vi "Configure Limit.vi"(4 "Lower Limit":dbl, 5 "Upper Limit":dbl, 6 "Enable Lower Limit (T: On)":bool=TRUE, 7 "Enable Upper Limit (T: On)":bool=TRUE, 8 "error in (no error)":errorcluster, 11 "VISA resource name":refnum<visa-resource-name>) -> (0 "error out":errorcluster, 3 "VISA resource name out":refnum<visa-resource-name>)   [LabVIEW 2019, in "Pendulum CNT90.lvlib"]
doc: "Turns On/Off the limit-monitoring calculations and the chacking against the lower or upper limit. And configures lower and upper limit."
uses:
  Pendulum CNT90.lvlib
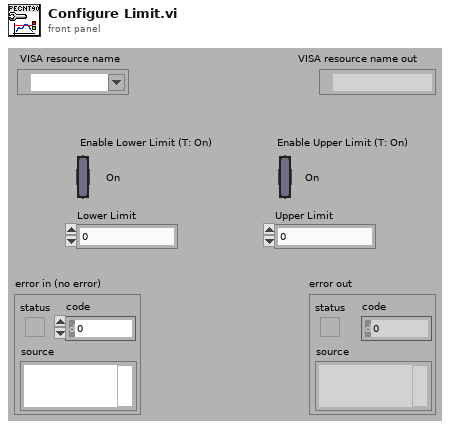
[diagram p1: front panel]
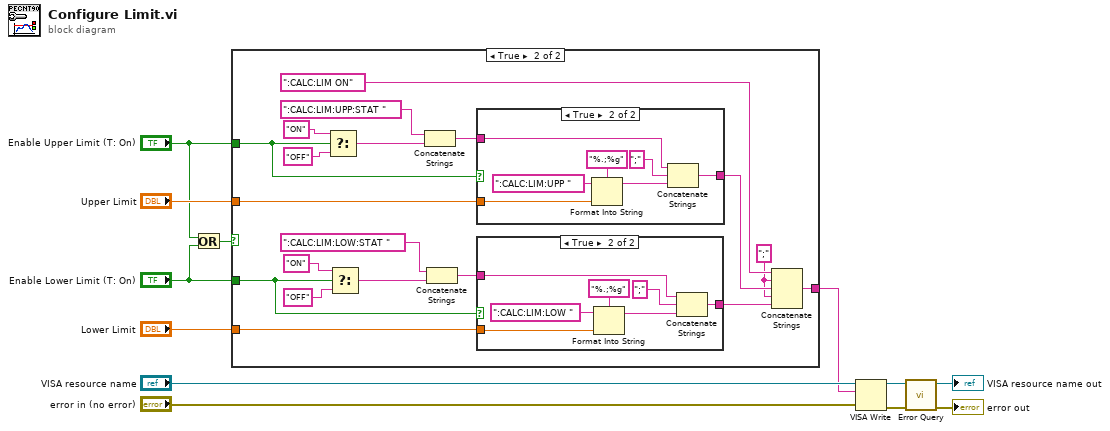
[diagram p0: block diagram]
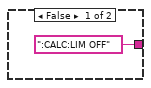
[diagram p2: hidden frame]
diagram:
  n1 = Or(x="Enable Upper Limit (T: On)", y="Enable Lower Limit (T: On)") -> (x .or. y?=w3:bool)
  n2 = case shown="True" w3 {
    tunnel: "Upper Limit" -> [_ w32]
    tunnel: "Lower Limit" -> [_ w31]
    tunnel: [":CALC:LIM OFF" w30] -> w4
    tunnel: "Enable Lower Limit (T: On)" -> [_ w20]
    tunnel: "Enable Upper Limit (T: On)" -> [_ w15]
    frame False {
    }
    frame True {
      w14 = ";" ("string")
      n3 = Select(t="ON", s=w15, f="OFF") -> (s? t:f=w24:string)
      n4 = Select(t="ON", s=w20, f="OFF") -> (s? t:f=w22:string)
      n5 = Concatenate Strings(":CALC:LIM:UPP:STAT ", w24) -> (w21:string)
      n6 = Concatenate Strings(":CALC:LIM:LOW:STAT ", w22) -> (w19:string)
      n7 = case shown="True" w15 {
        tunnel: w32 -> [_ w46]
        tunnel: w21 -> [w41 w44]
        tunnel: [w41 w42] -> w18
        frame False {
        }
        frame True {
          n8 = Format Into String(format string="%.;%g", initial string=":CALC:LIM:UPP ", w46) -> (resulting string=w45:string)  [unwired: 1 in, 1 out]
          n9 = Concatenate Strings(w44, ";" ("string"), w45) -> (w42:string)
        }
      }
      n10 = case shown="True" w20 {
        tunnel: w31 -> [_ w38]
        tunnel: w19 -> [w33 w36]
        tunnel: [w33 w34] -> w17
        frame False {
        }
        frame True {
          n11 = Format Into String(format string="%.;%g", initial string=":CALC:LIM:LOW ", w38) -> (resulting string=w37:string)  [unwired: 1 in, 1 out]
          n12 = Concatenate Strings(w36, ";" ("string"), w37) -> (w34:string)
        }
      }
      n13 = Concatenate Strings(":CALC:LIM ON", w14, w18, w14, w17) -> (w30:string)
    }
  }
  n14 = VISA Write(VISA resource name="VISA resource name", write buffer=w4, error in (no error)="error in (no error)") -> (VISA resource name out=w10:refnum<visa-resource-name>, error out=w7:errorcluster)  [unwired: 1 out]
  n15 = call "Error Query.vi"("error in (no error)"=w7, "VISA resource name"=w10) -> ("error out"=→"error out":errorcluster, "VISA resource name out"=→"VISA resource name out":refnum<visa-resource-name>)  [unwired: 6 in, 2 out]
